vi "createStyle.vi"(8 "error in (no error)":errorcluster, 10 "Style":refnum<class "Style.lvclass">, 11 "Section in":refnum<k24>) -> (0 "error out":errorcluster, 3 "Section out":refnum<k24>)   [LabVIEW 2017, in "LabVIEW NPOI.lvlib" / "xwpfWriter.lvclass"]
uses:
  xwpfWriter.lvclass
  Styles/Style/Style.lvclass
  C:/Users/Neo/Desktop/Dev_Tools_BR/LabVIEW_NPOI/lib/NPOI 2.1.1/NPOI.OOXML.dll
  lib/NPOI 2.1.1/NPOI.OOXML.dll
  Styles/Style/Get Color (Hex).vi
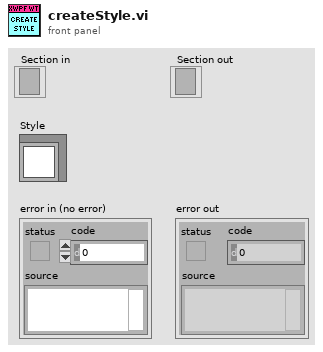
[diagram p1: front panel]
types:
  T1 = typedef "Styles.lvlib/Underline--ring.ctl" = i32
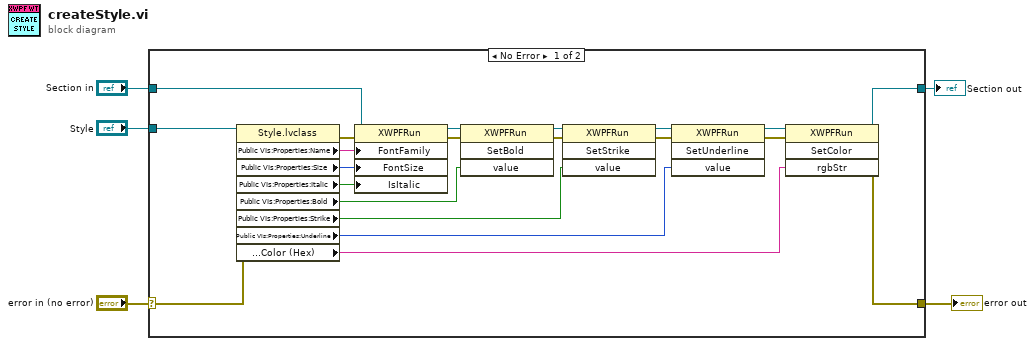
[diagram p0: block diagram]
diagram:
  n1 = case shown="No Error" "error in (no error)" {
    selector: "error in (no error)" -> [w25 w28]
    tunnel: [w7 w28] -> w4
    tunnel: "Style" -> [w26 _]
    tunnel: "Section in" -> [w24 w27]
    tunnel: [w6 w27] -> w1
    frame No Error {
      n2 = property class="Style.lvclass"(reference=w26, error in=w25) -> (error out=w8:errorcluster, "Public VIs:Properties:Name"=w20:string, "Public VIs:Properties:Size"=w19:i32, "Public VIs:Properties:Italic"=w18:bool, "Public VIs:Properties:Bold"=w17:bool, "Public VIs:Properties:Strike"=w16:bool, "Public VIs:Properties:Underline"=w15:T1, "Public VIs:Properties:Color (Hex)"=w13:string)  [unwired: 1 out]
      n3 = property class="XWPFRun"(reference=w24, error in=w8, "FontFamily"=w20, "FontSize"=w19, "IsItalic"=w18) -> (reference out=w23:refnum<k24>, error out=w12:errorcluster)
      n4 = invoke class="XWPFRun" method="SetBold"(reference=w23, error in=w12, "value"=w17) -> (reference out=w22:refnum<k24>, error out=w11:errorcluster)  [unwired: 1 in, 2 out]
      n5 = invoke class="XWPFRun" method="SetStrike"(reference=w22, error in=w11, "value"=w16) -> (reference out=w21:refnum<k24>, error out=w10:errorcluster)  [unwired: 1 in, 2 out]
      n6 = invoke class="XWPFRun" method="SetUnderline"(reference=w21, error in=w10, "value"=w15) -> (reference out=w14:refnum<k24>, error out=w9:errorcluster)  [unwired: 1 in, 2 out]
      n7 = invoke class="XWPFRun" method="SetColor"(reference=w14, error in=w9, "rgbStr"=w13) -> (reference out=w6:refnum<k24>, error out=w7:errorcluster)  [unwired: 1 in, 2 out]
    }
    frame Error {
    }
  }
  "error out" <- w4
  "Section out" <- w1
